vi "Determine Block Rotation.vi"(7 "Show line?":bool, 8 "error in (no error)":errorcluster, 11 "Image in":T2) -> (0 "error out":errorcluster, 1 "Straight Edges":T4(array[cluster]) {"Point2 (Real-World)"."Y" format="%.2f"; "Point2 (Real-World)"."X" format="%.2f"; "Point1 (Real-World)"."Y" format="%.2f"; "Point1 (Real-World)"."X" format="%.2f"; "Point2 (Pixels)"."Y" format="%.2f"; "Point2 (Pixels)"."X" format="%.2f"; "Point1 (Pixels)"."Y" format="%.2f"; "Point1 (Pixels)"."X" format="%.2f"}, 2 "Angle (Pixel)":dbl, 3 "Image out":T2)   [LabVIEW 2012]
uses:
  <vilib>/vision/Image Controls.llb/IMAQ Image.ctl
  <vilib>/vision/NI_Vision_Development_Module.lvlib
panel:
  in  "Edge Options":T1={"Edge Polarity"=0, "Kernel Size"=13, "Width"=1, "Minimum Edge Strength"=1.0, "Interpolation Type"=enum."Zero Order", "Data Processing Method"=enum."Average"} {"Edge Polarity" items=["All Edges", "Rising Edges", "Falling Edges"]}
  in  "Line Options":T3={"Number of Lines"=1, "Type"=enum."First Edge Rake", "Min. Score"=0.0, "Max. Score"=1024.0, "Orientation"=0.0, "Angle Range"=45.0, "Angle Tolerance"=1.0, "Step Size"=20, "Min. SNR (db)"=5.0, "Min. Points (%)"=25.0, "Hough Iterations"=5}
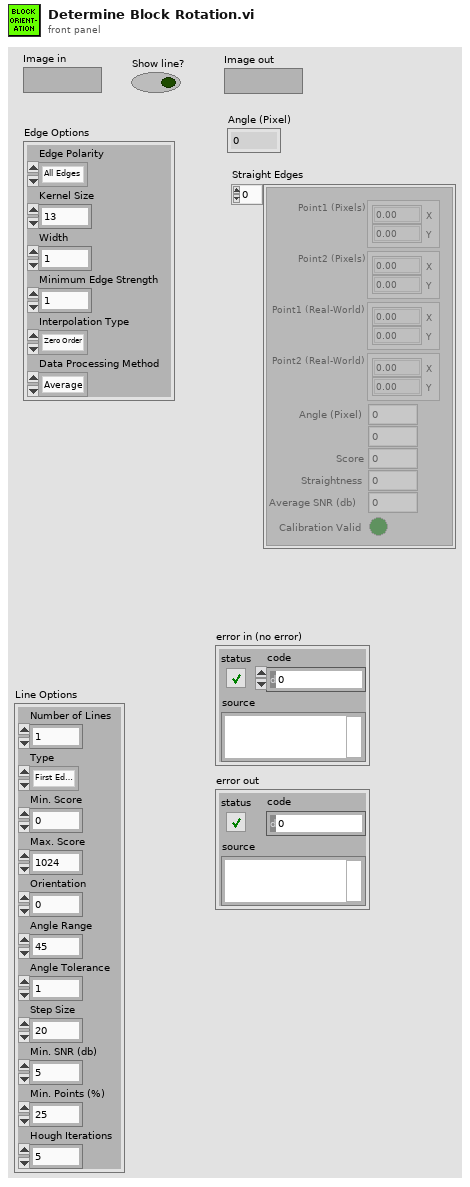
[diagram p1: front panel]
types:
  T1 = cluster{"Edge Polarity":u32, "Kernel Size":u32, "Width":u32, "Minimum Edge Strength":sgl, "Interpolation Type":enum32{"Zero Order", "Bilinear", "Quadratic", "Cubic", "Bilinear Fixed"}, "Data Processing Method":enum32{"Average", "Median"}}
  T2 = typedef "IMAQ Image.ctl" = refnum<image>
  T3 = cluster{"Number of Lines":i32, "Type":enum32{"First Edge Rake", "Best Edge Rake", "Hough Edge Rake", "First Edge Projection", "Best Edge Projection"}, "Min. Score":dbl, "Max. Score":dbl, "Orientation":dbl, "Angle Range":dbl, "Angle Tolerance":dbl, "Step Size":u32, "Min. SNR (db)":dbl, "Min. Points (%)":dbl, "Hough Iterations":i32}
  T4 = cluster{"Point1 (Pixels)":cluster{"X":sgl, "Y":sgl}, "Point2 (Pixels)":cluster{"X":sgl, "Y":sgl}, "Point1 (Real-World)":cluster{"X":sgl, "Y":sgl}, "Point2 (Real-World)":cluster{"X":sgl, "Y":sgl}, "Angle (Pixel)":dbl, "Angle (Real-World)":dbl, "Score":dbl, "Straightness":dbl, "Average SNR (db)":dbl, "Calibration Valid":bool}[]
  T5 = cluster{"Global Rectangle":i32[], "Contours":cluster{"ID":enum32{"External", "Internal"}, "Type":u32, "Coordinates":i32[]}[]}
  T6 = cluster{"Point1 (Pixels)":cluster{"X":sgl, "Y":sgl}, "Point2 (Pixels)":cluster{"X":sgl, "Y":sgl}, "Point1 (Real-World)":cluster{"X":sgl, "Y":sgl}, "Point2 (Real-World)":cluster{"X":sgl, "Y":sgl}, "Angle (Pixel)":dbl, "Angle (Real-World)":dbl, "Score":dbl, "Straightness":dbl, "Average SNR (db)":dbl, "Calibration Valid":bool}
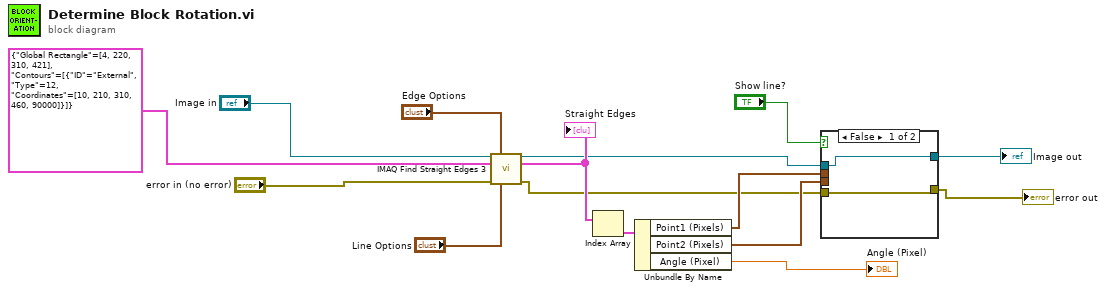
[diagram p0: block diagram]
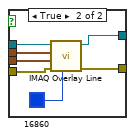
[diagram p2: hidden frame]
diagram:
  n1 = call "IMAQ Find Straight Edges 3"("Image"="Image in", "Edge Options"="Edge Options", "ROI Descriptor"=T5 {"Global Rectangle"=[4, 220, 310, 421], "Contours"=[{"ID"=enum."External", "Type"=12, "Coordinates"=[10, 210, 310, 460, 90000]}]}, "error in (no error)"="error in (no error)", "Line Options"="Line Options") -> ("Image (duplicate)"=w10:T2, "Straight Edges"=w12:T4, "error out"=w9:errorcluster)  [unwired: 6 in, 2 out]
  "Straight Edges" <- w12
  n2 = Index Array(array=w12) -> (element=w13:T6)  [unwired: 1 in]
  n3 = Unbundle By Name(w13) -> ("Point1 (Pixels)"=w14:cluster{"X":sgl, "Y":sgl}, "Point2 (Pixels)"=w15:cluster{"X":sgl, "Y":sgl}, "Angle (Pixel)"=→"Angle (Pixel)":dbl)
  n4 = case shown="False" "Show line?" {
    tunnel: w15 -> [_ w24]
    tunnel: w14 -> [_ w23]
    tunnel: [w16 w21] -> w11
    tunnel: w10 -> [w17 w20]
    tunnel: w9 -> [w16 w19]
    tunnel: [w17 w18] -> w5
    frame False {
    }
    frame True {
      n5 = call "IMAQ Overlay Line"("Color"=u32 16860, "error in (no error)"=w19, "End Point"=w24, "Start Point"=w23, "Image"=w20) -> ("error out"=w21:errorcluster, "Image Out"=w18:T2)  [unwired: 5 in]
    }
  }
  "error out" <- w11
  "Image out" <- w5
